vi "get total.vi"(10 "Tree":T1) -> (2 "Tree 2":T1)   [LabVIEW 2020]
uses:
  tree--cluster.ctl
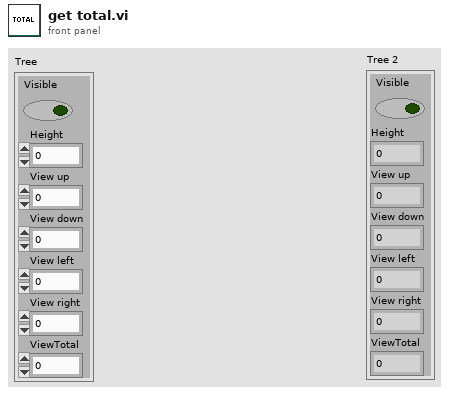
[diagram p1: front panel]
types:
  T1 = typedef "tree--cluster.ctl" = cluster{"Visible":bool, "Height":i32, "View up":i32, "View down":i32, "View left":i32, "View right":i32, "ViewTotal":i32}
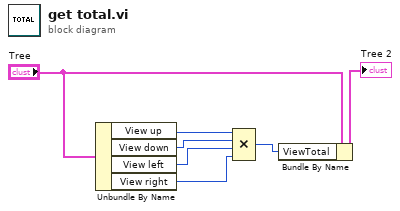
[diagram p0: block diagram]
diagram:
  n1 = Unbundle By Name("Tree") -> ("View up"=w7:i32, "View down"=w6:i32, "View left"=w5:i32, "View right"=w4:i32)
  n2 = Compound Arithmetic op=MULTIPLY(w7, w6, w5, w4) -> (w2:i32)
  n3 = Bundle By Name(cluster="Tree", "ViewTotal"=w2) -> (→"Tree 2":T1)
